vi "Process-error.vi"(8 "error in (no error)":errorcluster, 11 "Data in":T1) -> (0 "error out":errorcluster, 3 "Data out":T1)   [LabVIEW 2013, in "PowderDeposition.lvlib" / "PD-Main.lvclass"]
uses:
  PD-Main.lvclass
  Object-reference.ctl
  <vilib>/Utility/error.llb/DialogType.ctl
  Communication/Sources/PD-Client.lvclass
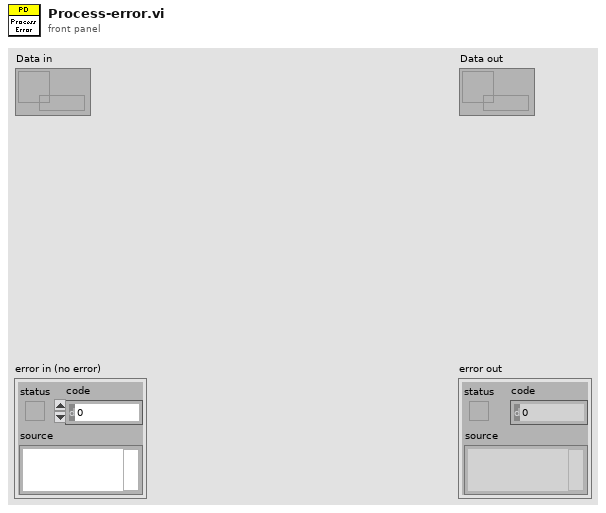
[diagram p1: front panel]
types:
  T1 = typedef "PowderDeposition.lvlib/PD-Main.lvclass/Object-reference.ctl" = refnum<data-value>
  T2 = typedef "DialogType.ctl" = u16
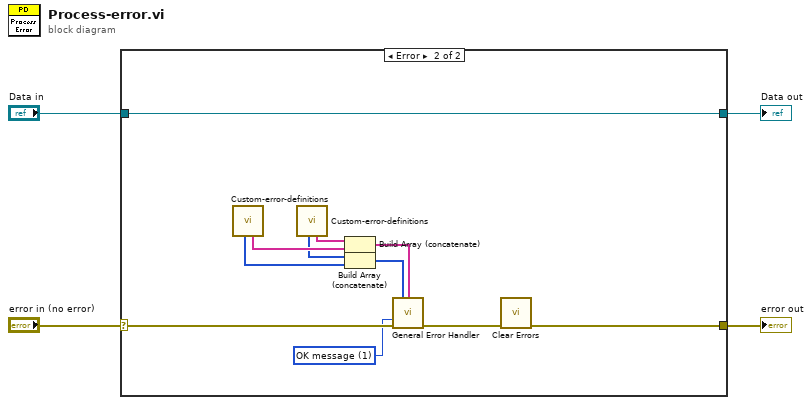
[diagram p0: block diagram]
diagram:
  n1 = case shown="Error" "error in (no error)" {
    selector: "error in (no error)" -> [w6 w17]
    tunnel: [w6 w14] -> w3
    tunnel: [w5 w16] -> w1
    tunnel: "Data in" -> [w5 w16]
    frame No Error {
    }
    frame Error {
      w13 = T2 1 items=["no dialog", "OK message", "continue or stop message", "OK message + warnings", "continue/stop + warnings"] ("type of dialog (OK msg:1)")
      n2 = call "Custom-error-definitions.vi"() -> ("Descriptions"=w11:string[], "Error codes"=w9:i32[])  [unwired: 9 in, 1 out]
      n3 = call "Custom-error-definitions.vi"() -> ("Descriptions"=w12:string[], "Error codes"=w10:i32[])  [unwired: 9 in, 1 out]
      n4 = Build Array (concatenate)(w12, w11) -> (w8:string[])
      n5 = Build Array (concatenate)(w10, w9) -> (w7:i32[])
      n6 = call <vilib>:"General Error Handler.vi"("[user-defined codes]"=w7, "[user-defined descriptions]"=w8, "type of dialog (OK msg:1)"=w13, "error in (no error)"=w17) -> ("error out"=w15:errorcluster)  [unwired: 7 in, 4 out]
      n7 = call <vilib>:"Clear Errors.vi"("error in (no error)"=w15) -> ("error out"=w14:errorcluster)  [unwired: 6 in]
    }
  }
  "error out" <- w3
  "Data out" <- w1
